vi "2D To 1D.vi"(11 "Pixel Data in":u32[][](array[numeric])) -> (3 "1D Pixel Data out":u32[](array[numeric]))   [LabVIEW 2020, in "3D (FPGA).lvlib"]
uses:
  3D (FPGA).lvlib
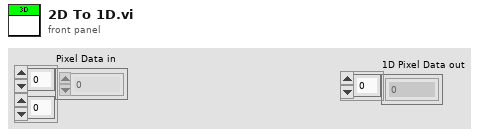
[diagram p1: front panel]
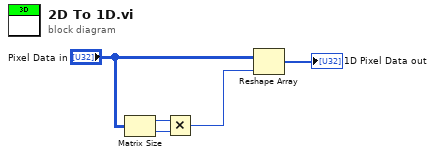
[diagram p0: block diagram]
diagram:
  n1 = Matrix Size(0:"Pixel Data in") -> (1:w4:i32, 2:w3:i32)
  n2 = Multiply(x=w4, y=w3) -> (x*y=w2:i32)
  n3 = Reshape Array("Pixel Data in", w2) -> (→"1D Pixel Data out":u32[])
